vi "Array - Read Age.vi"(8 "error in (no error)":errorcluster, 11 "Input Array":refnum<class "myClass.lvclass">[](array[class])) -> (0 "error out":errorcluster, 2 "Ages":dbl[](array[numeric]), 3 "Output Array":refnum<class "myClass.lvclass">[](array[class]))   [LabVIEW 2010]
uses:
  ClassDefinitions/SimpleClassWithProperties/myClass.lvclass
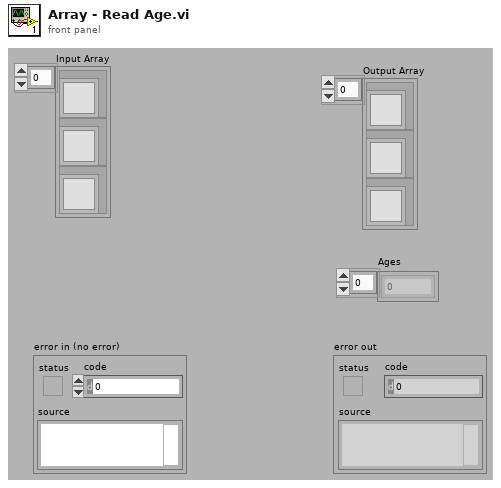
[diagram p1: front panel]
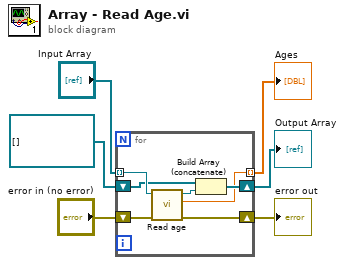
[diagram p0: block diagram]
diagram:
  n1 = for {
    tunnel: "Input Array" -> [w13] mode=indexing
    shift-right: [w10] -> w4
    shift-left: refnum<class "myClass.lvclass">[] [] ("Input Array") -> [w12]
    shift-right: [w9] -> w2
    shift-left: "error in (no error)" -> [w8]
    tunnel: [w7] -> w1 mode=indexing
    n2 = call-dynamic "Read age.vi"("error in (no error)"=w8, "myClass in"=w13) -> ("error out"=w9:errorcluster, "age"=w7:dbl, "myClass out"=w11:refnum<class "myClass.lvclass">)  [unwired: 7 in]
    n3 = Build Array (concatenate)(w12, w11) -> (w10:refnum<class "myClass.lvclass">[])
  }
  "Output Array" <- w4
  "error out" <- w2
  "Ages" <- w1
